vi "PH_GUI.set waveform chart GUI object.vi"(2 "WaveformChart in":refnum<vi>, 3 "Double":dbl, 5 "error in (no error)":errorcluster) -> (19 "error out":errorcluster)   [LabVIEW 2014, in "PH_Common.lvlib"]
uses:
  PH_Common.lvlib
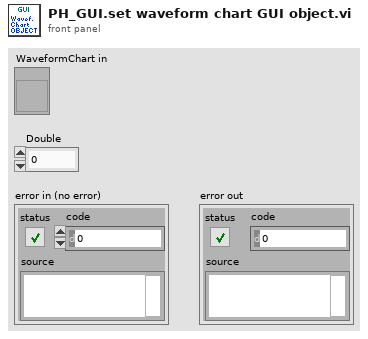
[diagram p1: front panel]
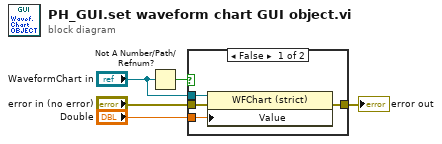
[diagram p0: block diagram]
diagram:
  n1 = Not A Number/Path/Refnum?(number/path/refnum="WaveformChart in") -> (NaN/Path/Refnum?=w1:bool)
  n2 = case shown="False" w1 {
    tunnel: "Double" -> [w9 _]
    tunnel: "error in (no error)" -> [w8 w10]
    tunnel: [w7 w10] -> w3
    tunnel: "WaveformChart in" -> [w6 _]
    frame False {
      n3 = property class="WFChart (strict)"(reference=w6, error in=w8, "Value"=w9) -> (error out=w7:errorcluster)  [unwired: 1 out]
    }
    frame True {
    }
  }
  "error out" <- w3
